vi "Get Item Name.vi"(8 "error in":errorcluster, 11 "Item Ref":T1 format="%.0x") -> (0 "error out":errorcluster, 2 "Name":string, 3 "Item Ref out":T1 format="%.0x")   [LabVIEW 2020, in "Communication Bus Template Scripting.lvlib"]
uses:
  <vilib>/NI VeriStand/Custom Device API/Custom Device Item Ref.ctl
  Communication Bus Template Scripting.lvlib
  <vilib>/NI VeriStand/Custom Device API/Custom Device API.lvlib
panel:
  in  "Name 2":string
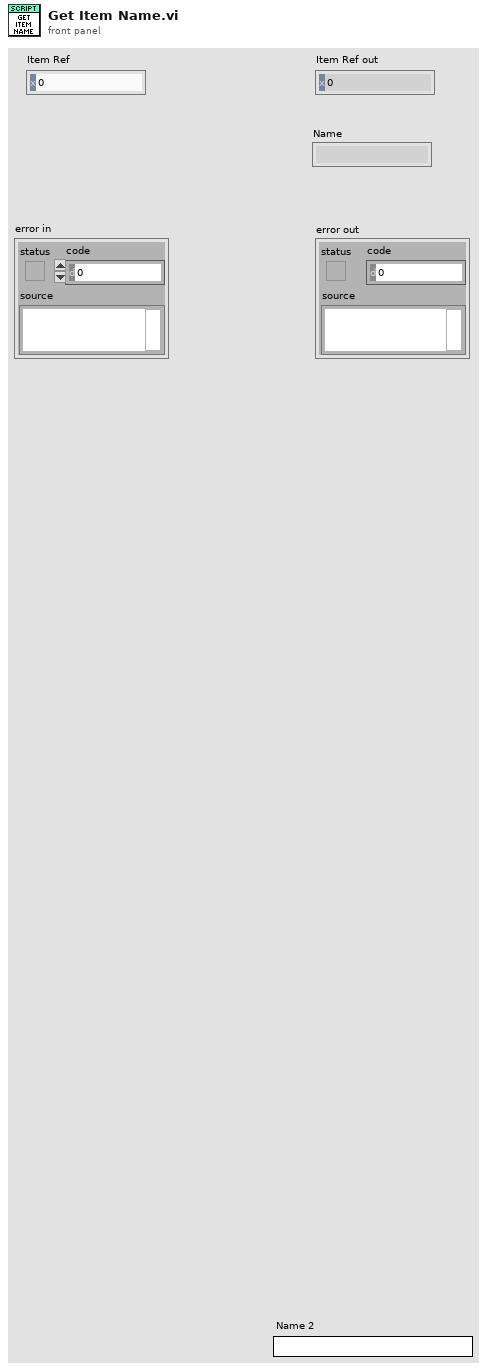
[diagram p1: front panel]
types:
  T1 = typedef "Custom Device API.lvlib/Custom Device Item Ref.ctl" = u64
  T2 = typedef "Custom Device API.lvlib/Custom Device Item Info.ctl" = cluster{"Name":string, "Is Channel":bool, "GUID":string, "Is Waveform":bool}
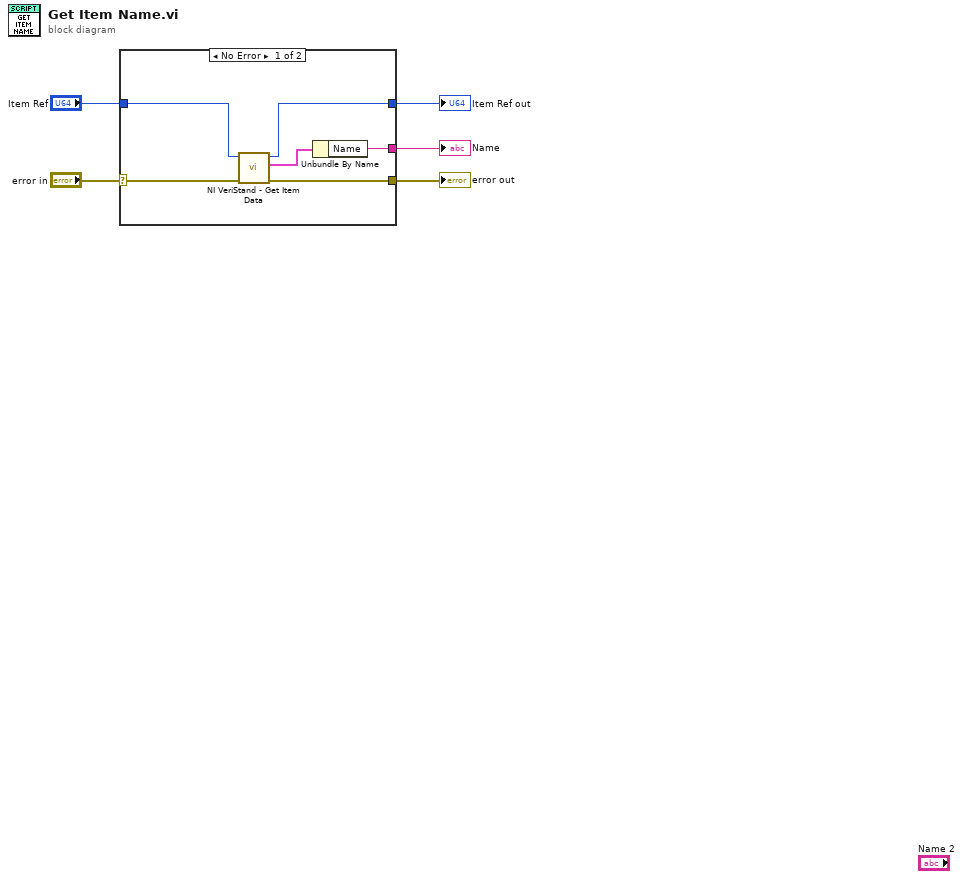
[diagram p0: block diagram]
diagram:
  n1 = case shown="No Error" "error in" {
    selector: "error in" -> [w10 w13]
    tunnel: [w9 w13] -> w2
    tunnel: "Item Ref" -> [w6 w12]
    tunnel: [w7 w12] -> w4
    tunnel: [w8 _] -> w5
    frame No Error {
      n2 = call <vilib>:"NI VeriStand - Get Item Data.vi"("error in (no error)"=w10, "Item Ref in"=w6) -> ("error out"=w9:errorcluster, "Item Info"=w11:T2, "Item Ref out"=w7:T1)  [unwired: 7 out]
      n3 = Unbundle By Name(w11) -> ("Name"=w8:string)
    }
    frame Error {
    }
  }
  "Name" <- w5
  "Item Ref out" <- w4
  "error out" <- w2
